vi "run.create.vi"(8 "error in":errorcluster, 9 "Start Time (now)":timestamp format="%<%x %.3X>T", 10 "Title":string, 11 "asset in":refnum<class "asset.lvclass">) -> (0 "error out":errorcluster, 2 "Run":refnum<class "Run.lvclass">, 3 "asset out":refnum<class "asset.lvclass">)   [LabVIEW 2020, in "asset.lvclass"]
uses:
  asset.lvclass
  Run/Run.lvclass
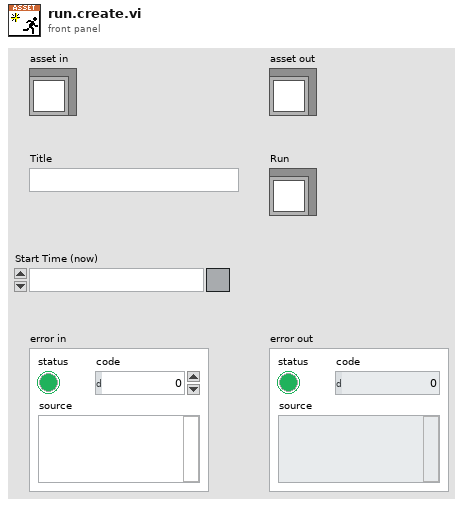
[diagram p1: front panel]
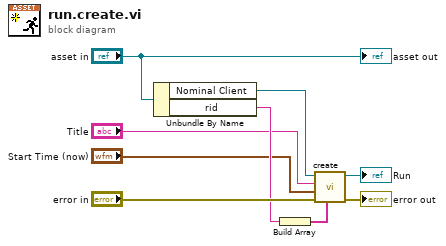
[diagram p0: block diagram]
diagram:
  n1 = Unbundle By Name("asset in") -> ("Nominal Client"=w9:refnum<class "Nominal Client.lvclass">, "rid"=w5:string)
  n2 = Build Array(w5) -> (w4:string[])
  n3 = call "create.vi"("Assets"=w4, "error in (no error)"="error in", "Start Time"="Start Time (now)", "Title"="Title", "Nominal Client"=w9) -> ("error out"=→"error out":errorcluster, "Run out"=→"Run":refnum<class "Run.lvclass">)  [unwired: 5 in]
  "asset out" <- "asset in"
